vi "Convert serial string to Eng vals.vi"(0 "Serial buffer string (excluding FrameChar)":string) -> (3 "Pressures":sgl[][](graph), 4 "Atmospheric pressure (mbar)":sgl, 6 "External thermistor temperature (deg C)":sgl, 8 "Env. sensor die temperature (deg C)":sgl, 10 "Relative humidity (%)":sgl, 13 "All vals":sgl[](array[numeric]), 14 "Gyration vector (deg / s)":sgl[](array[numeric]), 15 "Acceleration vector (g)":sgl[](array[numeric]))   [LabVIEW 2017]
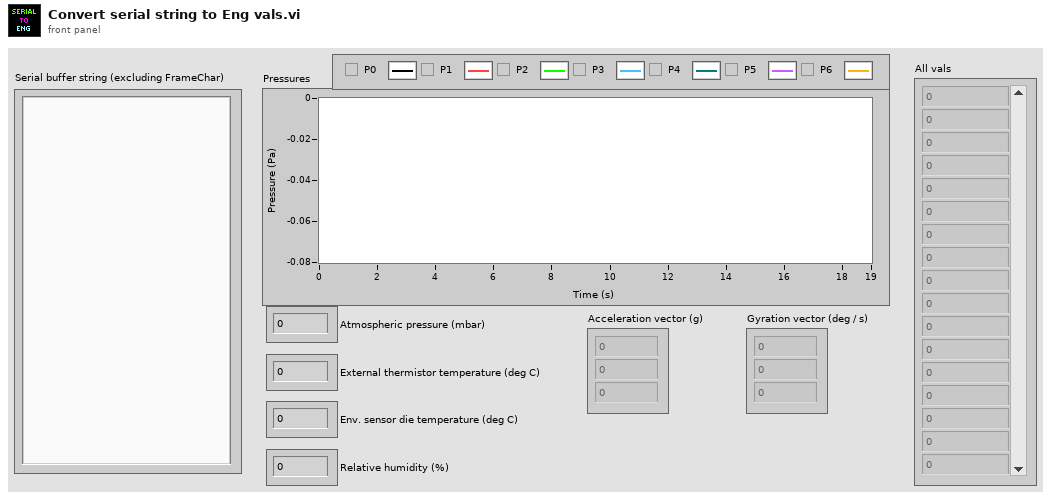
[diagram p1: front panel]
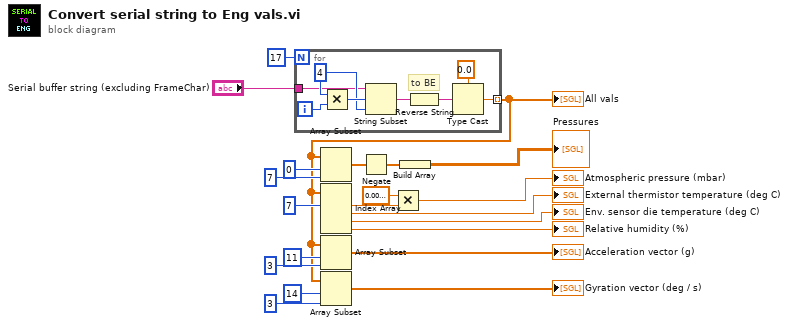
[diagram p0: block diagram]
diagram:
  n1 = for {
    N: 17 -> [_]
    tunnel: [w23] -> w3 mode=indexing
    tunnel: "Serial buffer string (excluding FrameChar)" -> [w22]
    i -> [w29]
    w27 = 4 ("x")
    # "to BE"
    n2 = Multiply(x=w27, y=w29) -> (x*y=w28:i32)
    n3 = String Subset(string=w22, offset (0)=w28, length (rest)=w27) -> (substring=w26:string)
    n4 = Reverse String(1:w26) -> (0:w25:string)
    n5 = Type Cast(type=sgl 0.0 ("byte count"), x=w25) -> (*(type *) &x=w23:sgl)
  }
  "All vals" <- w3
  n6 = Array Subset(array=w3, index=0, length=7) -> (w17:sgl[])
  n7 = Index Array(array=w3, index #1=7 ("index")) -> (element #1=w15:sgl, element #2=→"External thermistor temperature (deg C)":sgl, element #3=→"Env. sensor die temperature (deg C)":sgl, element #4=→"Relative humidity (%)":sgl)  [unwired: 3 in]
  n8 = Array Subset(array=w3, index=11, length=3) -> (→"Acceleration vector (g)":sgl[])
  n9 = Array Subset(array=w3, index=14, length=3) -> (→"Gyration vector (deg / s)":sgl[])
  n10 = Negate(x=w17) -> (-x=w1:sgl[])
  n11 = Multiply(x=sgl 0.01, y=w15) -> (x*y=→"Atmospheric pressure (mbar)":sgl)
  n12 = Build Array(w1) -> (→"Pressures":sgl[][])
